vi "Add Initialization Block Diagram Content.vi"(8 "error in (no error)":errorcluster, 10 "Init":T1, 11 "IO Class in":refnum<class "Signal.lvclass">) -> (0 "error out":errorcluster, 3 "IO Class out":refnum<class "Signal.lvclass">)   [LabVIEW 2015, in "Signal.lvclass"]
uses:
  Signal.lvclass
  Loop/Block Diagram/Init.Refs.ctl
  <vilib>/Utility/miscctls.llb/LVPointTypeDef.ctl
  Loop/Block Diagram/Block Diagram.lvclass
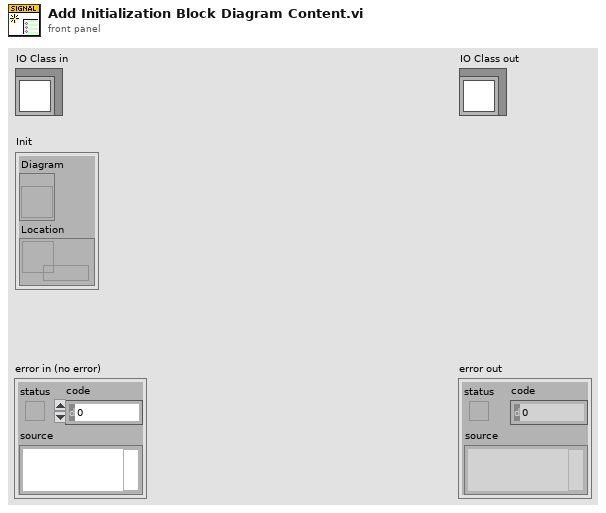
[diagram p1: front panel]
types:
  T1 = typedef "Block Diagram.lvclass/Init.Refs.ctl" = cluster{"Diagram":refnum<vi>, "Location":refnum<data-value>}
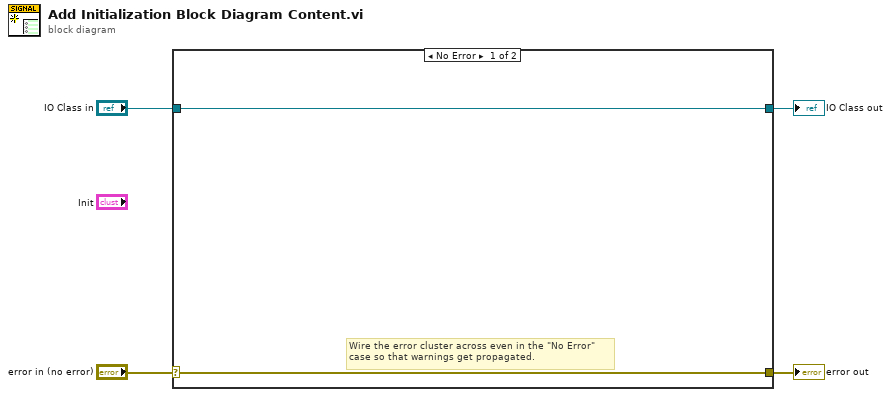
[diagram p0: block diagram]
diagram:
  n1 = case shown="No Error" "error in (no error)" {
    selector: "error in (no error)" -> [w5 w8]
    tunnel: [w5 w8] -> w3
    tunnel: [w6 w7] -> w1
    tunnel: "IO Class in" -> [w6 w7]
    frame No Error {
      # "Wire the error cluster across even in the \"No Error\"\ncase so that warnings get propagated."
    }
    frame Error {
    }
  }
  "error out" <- w3
  "IO Class out" <- w1
